vi "Get Client Command Specifier.vi"(8 "error in":errorcluster, 11 "CANopen Request in":refnum<class "CANopen Request Message.lvclass">) -> (0 "error out":errorcluster, 2 "Client Command Specifier":T1, 3 "CANopen Request out":refnum<class "CANopen Request Message.lvclass">)   [LabVIEW 2024, in "CANopen Master.lvlib" / "CANopen Request Message.lvclass"]
uses:
  CANopen Request Message.lvclass
  CANopen Request Message.lvclass/CANopen Request Message.ctl
  CANopen/Client Command Specifier.ctl
  CANopen Message/CANopen Message.lvclass
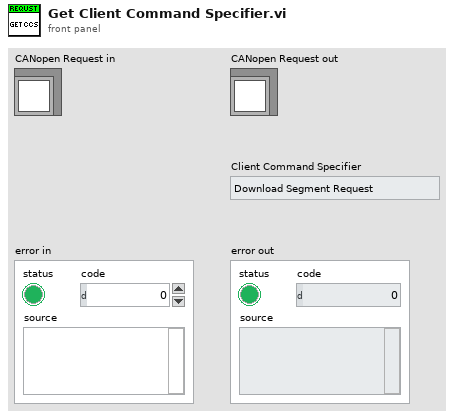
[diagram p1: front panel]
types:
  T1 = typedef "CANopen Master.lvlib/CANopen Request Message.lvclass/Client Command Specifier.ctl" = enum8{"Download Segment Request", "Initiate Download Request", "Initiate Upload Request", "Upload Segment Request", "Heartbeat", "UNKNOWN", "Block Download"}
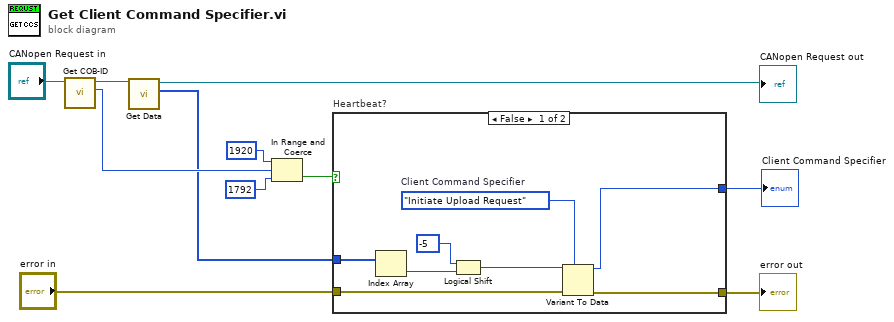
[diagram p0: block diagram]
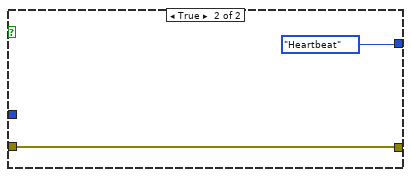
[diagram p2: hidden frame]
diagram:
  n1 = call "Get COB-ID.vi"("CANopen Message in"="CANopen Request in") -> ("COB-ID"=w6:u32, "CANopen Message out"=w9:refnum<class "CANopen Request Message.lvclass">)  [unwired: 9 in]
  n2 = call "Get Data.vi"("CANopen Message in"=w9) -> ("Data"=w5:u8[], "CANopen Message out"=→"CANopen Request out":refnum<class "CANopen Request Message.lvclass">)  [unwired: 9 in]
  n3 = In Range and Coerce(upper limit=u32 1920 ("x"), x=w6, lower limit=u32 1792 ("x")) -> (In Range?=w1:bool)  [unwired: 1 out]
  n4 = case "Heartbeat?" shown="False" w1 {
    tunnel: w5 -> [w19 _]
    tunnel: [w12 Client_Command_Specifier."Heartbeat" ("Msg-Type")] -> w2
    tunnel: "error in" -> [w14 w20]
    tunnel: [w13 w20] -> w3
    frame False {
      w16 = Client_Command_Specifier."Initiate Upload Request"  # Client Command Specifier
      n5 = Index Array(array=w19) -> (element=w17:u8)  [unwired: 1 in]
      n6 = Logical Shift(y=-5 ("x"), x=w17) -> (x << y=w15:u8)
      n7 = Variant To Data(error in=w14, type=w16, Variant=w15) -> (data=w12:T1, error out=w13:errorcluster)
    }
    frame True {
    }
  }
  "Client Command Specifier" <- w2
  "error out" <- w3
